vi "conversion_deg_to_rad.vi"(1 "Angle (deg)":dbl) -> (0 "Angle (rad)":dbl)   [LabVIEW 2021]
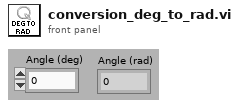
[diagram p1: front panel]
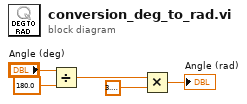
[diagram p0: block diagram]
diagram:
  n1 = Divide(x="Angle (deg)", y=180.0) -> (x/y=w4:dbl)
  n2 = Multiply(x=w4, y=3.141592653589793) -> (x*y=→"Angle (rad)":dbl)
